vi "Version 1_Read Totalizer Options.vi"(7 "Address (A)":string="A", 8 "error in":errorcluster, 11 "VISA Session In":refnum<visa-resource-name>="Alicat") -> (0 "error out":errorcluster, 1 "Totalizer Setup":T1, 3 "VISA Session Out":refnum<visa-resource-name>)   [LabVIEW 2016]
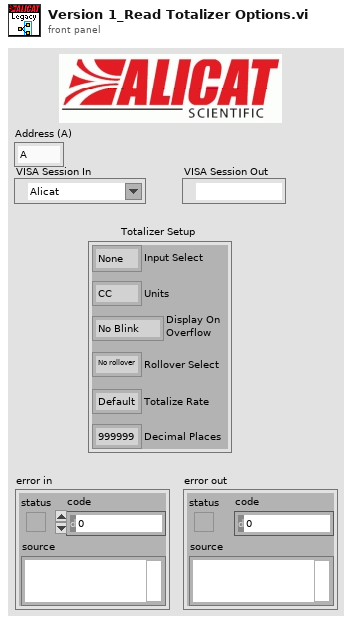
[diagram p1: front panel]
types:
  T1 = cluster{"Input Select":enum8{"None", "Volume", "Mass"}, "Units":enum8{"CC", "uL", "L", "CI", "CF", "CM", "GAL", "mL", "uP", "Lbs", "unknown (10)", "unknown (11)", "unknown (12)", "unknown (13)", "unknown (14)", "unknown (15)", "SCC", "SuL", "SL", "SCI", "SCF", "NCM", "Grams", "Kg", "lbs", "mg", "SCM", "smL", "KSCF"}, "Display On \nOverflow":enum32{"No Blink", "Blink"}, "Rollover Select":enum8{"No rollover", "Rollover with error on overflow", "Rollover with no error on overflow"}, "Totalize Rate":enum8{"Default", "Use R84", "Enable pulse out", "Breath", "Hide totalizer"}, "Decimal Places":enum8{"999999", "99999.9", "9999.99", "999.999", "99.9999", "099.9999", "0099.9999", "00099.9999"}}
  T2 = cluster{"Input Select":enum8{"None", "Volume", "Mass"}, "Units":enum8{"CC", "uL", "L", "CI", "CF", "CM", "GAL", "mL", "uP", "Lbs", "unknown (10)", "unknown (11)", "unknown (12)", "unknown (13)", "unknown (14)", "unknown (15)", "SCC", "SuL", "SL", "SCI", "SCF", "NCM", "Grams", "Kg", "lbs", "mg", "SCM", "smL", "KSCF"}, "Display On Overflow":enum32{"No Blink", "Blink"}, "Rollover Select":enum8{"No rollover", "Rollover with error on overflow", "Rollover with no error on overflow"}, "Totalize Rate":enum8{"Default", "Use R84", "Enable pulse out", "Breath", "Hide totalizer"}, "Decimal Places":enum8{"999999", "99999.9", "9999.99", "999.999", "99.9999", "099.9999", "0099.9999", "00099.9999"}}
  T3 = enum8{"CC", "uL", "L", "CI", "CF", "CM", "GAL", "mL", "uP", "Lbs", "unknown (10)", "unknown (11)", "unknown (12)", "unknown (13)", "unknown (14)", "unknown (15)", "SCC", "SuL", "SL", "SCI", "SCF", "NCM", "Grams", "Kg", "lbs", "mg", "SCM", "smL", "KSCF"}
  T4 = enum8{"No rollover", "Rollover with error on overflow", "Rollover with no error on overflow"}
  T5 = enum8{"Default", "Use R84", "Enable pulse out", "Breath", "Hide totalizer"}
  T6 = enum8{"999999", "99999.9", "9999.99", "999.999", "99.9999", "099.9999", "0099.9999", "00099.9999"}
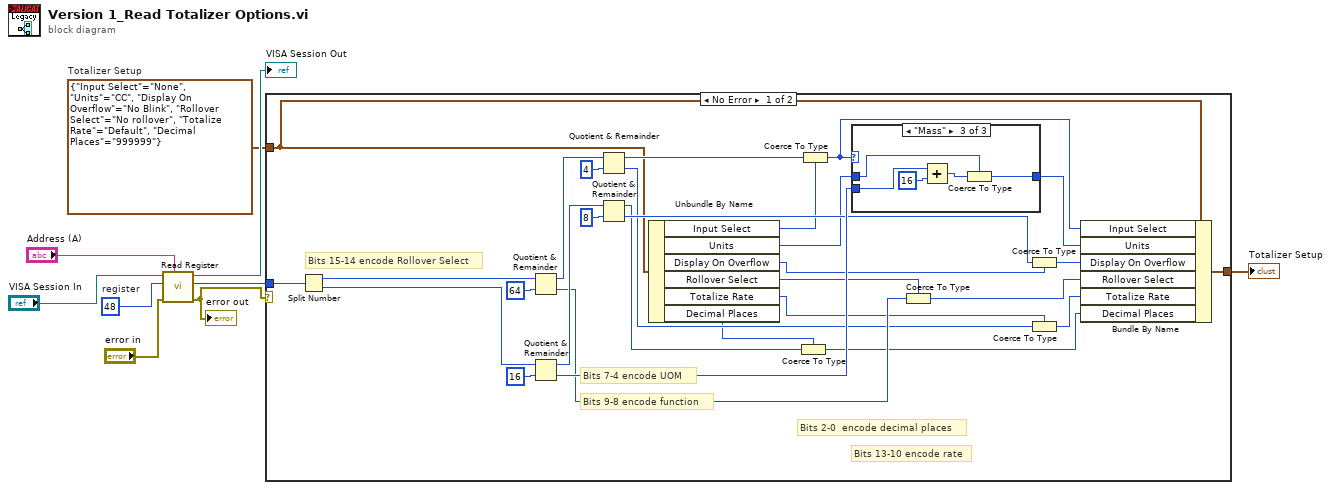
[diagram p0: block diagram]
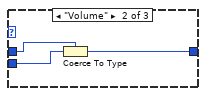
[diagram p3: hidden frame]
diagram:
  w2 = T2 {"Input Select"=enum."None", "Units"=enum."CC", "Display On Overflow"=enum."No Blink", "Rollover Select"=enum."No rollover", "Totalize Rate"=enum."Default", "Decimal Places"=enum."999999"}  # Totalizer Setup
  w9 = u16 48  # register
  n1 = call "Read Register.vi"("Unit ID (A)"="Address (A)", "error in"="error in", "Register address"=w9, "VISA Session In"="VISA Session In") -> ("error out"=w4:errorcluster, "Register Value (I32)"=w3:i32, "VISA Session Out"=→"VISA Session Out":refnum<visa-resource-name>)  [unwired: 5 in]
  "error out" <- w4
  n2 = case shown="No Error" w4 {
    tunnel: w3 -> [w38 _]
    tunnel: w2 -> [w16 w48]
    tunnel: [w17 w48] -> w1
    frame No Error {
      # "Bits 13-10 encode rate"
      # "Bits 15-14 encode Rollover Select"
      # "Bits 9-8 encode function"
      # "Bits 7-4 encode UOM"
      # "Bits 2-0  encode decimal places"
      n3 = Split Number(x=w38) -> (hi(x)=w26:u16, lo(x)=w37:u16)
      n4 = Quotient & Remainder(x=w26, y=u8 64) -> (x-y*floor(x/y)=w27:u16, floor(x/y)=w25:u16)
      n5 = Quotient & Remainder(x=w37, y=u8 16) -> (x-y*floor(x/y)=w32:u16, floor(x/y)=w34:u16)
      n6 = Quotient & Remainder(x=w27, y=u8 4) -> (x-y*floor(x/y)=w31:u16, floor(x/y)=w24:u16)
      n7 = Quotient & Remainder(x=w32, y=u8 8) -> (x-y*floor(x/y)=w29:u16, floor(x/y)=w30:u16)
      n8 = Unbundle By Name(w16) -> ("Input Select"=w15:enum8{"None", "Volume", "Mass"}, "Units"=w12:T3, "Display On Overflow"=w13:enum32{"No Blink", "Blink"}, "Rollover Select"=w10:T4, "Totalize Rate"=w11:T5, "Decimal Places"=w14:T6)
      n9 = Coerce To Type(0:w29, 1:w14) -> (2:w18:T6)
      n10 = Coerce To Type(0:w31, 1:w15) -> (2:w23:enum8{"None", "Volume", "Mass"})
      n11 = case shown="\"Mass\"" w23 {
        tunnel: w34 -> [_ w41 w47]
        tunnel: [w39 w40 w43] -> w22
        tunnel: w12 -> [w39 w42 w44]
        frame "None" {
        }
        frame "Volume" {
          n12 = Coerce To Type(0:w41, 1:w42) -> (2:w40:T3)
        }
        frame "Mass" {
          n13 = Add(x=w47, y=u8 16) -> (x+y=w45:u16)
          n14 = Coerce To Type(0:w45, 1:w44) -> (2:w43:T3)
        }
      }
      n15 = Coerce To Type(0:w25, 1:w10) -> (2:w20:T4)
      n16 = Coerce To Type(0:w30, 1:w13) -> (2:w21:enum32{"No Blink", "Blink"})
      n17 = Coerce To Type(0:w24, 1:w11) -> (2:w19:T5)
      n18 = Bundle By Name(cluster=w16, "Input Select"=w23, "Units"=w22, "Display On Overflow"=w21, "Rollover Select"=w20, "Totalize Rate"=w19, "Decimal Places"=w18) -> (w17:T2)
    }
    frame Error {
    }
  }
  "Totalizer Setup" <- w1
